vi "Write Port.vi"(8 "error in (no error)":errorcluster, 10 "port":u16, 11 "TCP in":refnum<class "TCP.lvclass">) -> (0 "error out":errorcluster, 3 "TCP out":refnum<class "TCP.lvclass">)   [LabVIEW 2019, in "TCP.lvclass"]
doc: "Property accessor for the TCP port."
uses:
  TCP.lvclass
  TCP.lvclass/TCP.ctl
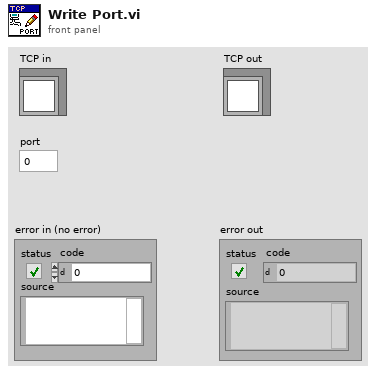
[diagram p1: front panel]
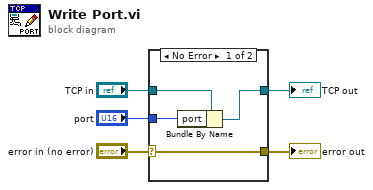
[diagram p0: block diagram]
diagram:
  n1 = case shown="No Error" "error in (no error)" {
    selector: "error in (no error)" -> [w6 w11]
    tunnel: "TCP in" -> [w9 w10]
    tunnel: [w8 w10] -> w4
    tunnel: "port" -> [w7 _]
    tunnel: [w6 w11] -> w1
    frame No Error {
      n2 = Bundle By Name(cluster=w9, "port"=w7) -> (w8:refnum<class "TCP.lvclass">)
    }
    frame Error {
    }
  }
  "error out" <- w1
  "TCP out" <- w4
